vi "Pointer producer consumer Manual Motor Controls.vi"(0 "Iteraction Counter":u32, 1 "loopback":bool, 5 "Input Array":bool[](array[boolean]), 6 "Impulse IN":i32, 8 "Reverse moving":bool, 9 "PA°":u16 max=359, 11 "PA Correction°":dbl min=-26.3 max=26.3 step=0.1 format="%#_3g", 13 "No. Impulses":u8, 14 "Modulo num":u8) -> (3 "get info?":bool, 4 "PA rounded":dbl, 10 "Output Number":i32, 12 "Impulses":bool, 15 "Impulse OUT":i32)   [LabVIEW 2014]
panel:
  out "PA real":dbl
  out "Array Code IN":u32
  out "Output Command":string
  out "Array Code OUT":u32
  out "HEX Out Cmd":string=" "
  in  "error in (no error)":errorcluster
  out "Down":bool
  out "Left":bool
  out "Up":bool
  out "Right":bool
  # "Autobalance"
  # "Array code after angle transposition"
  # "Loopback"
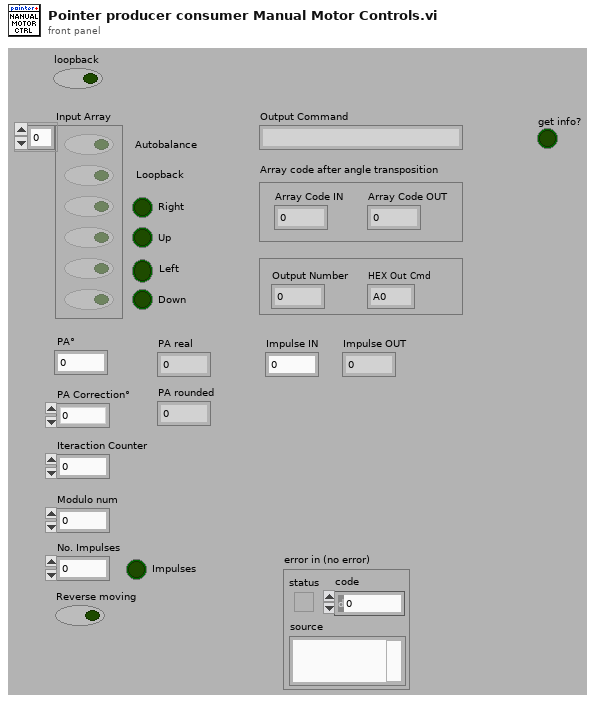
[diagram p1: front panel]
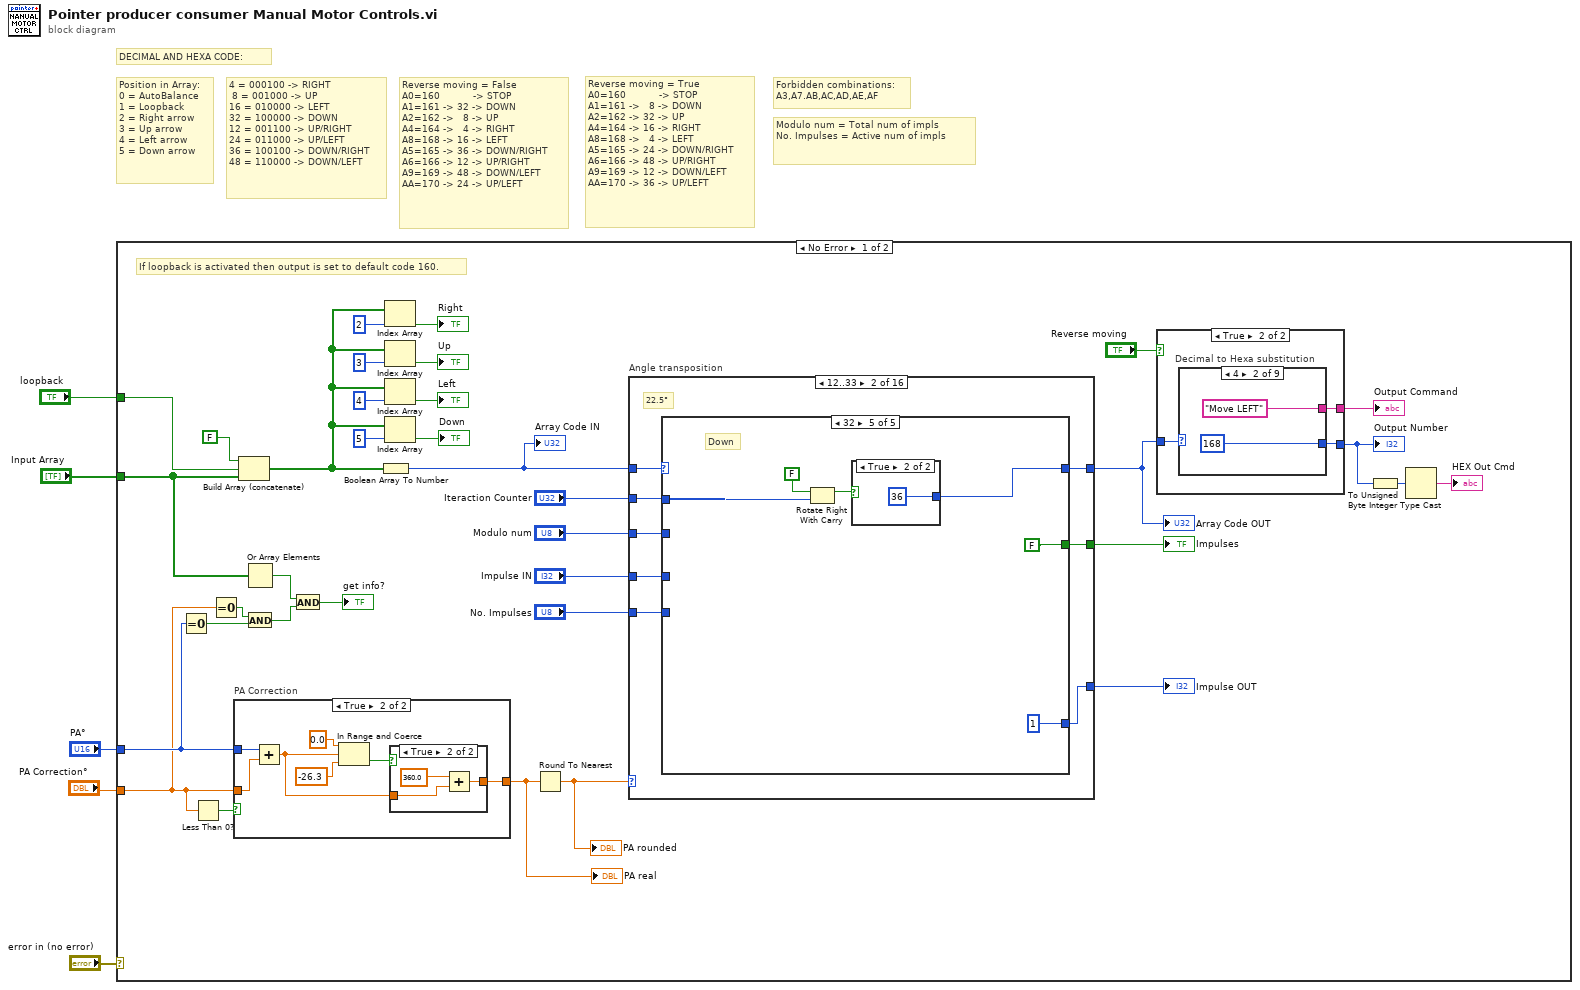
[diagram p0: block diagram]
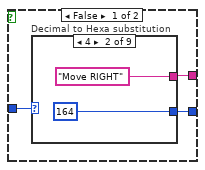
[diagram p2: hidden frame]
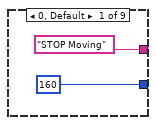
[diagram p3: hidden frame]
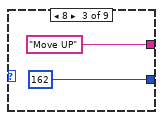
[diagram p4: hidden frame]
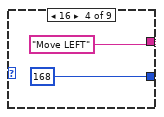
[diagram p5: hidden frame]
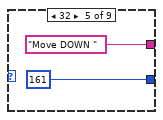
[diagram p6: hidden frame]
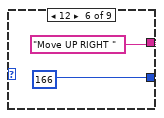
[diagram p7: hidden frame]
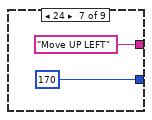
[diagram p8: hidden frame]
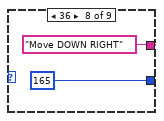
[diagram p9: hidden frame]
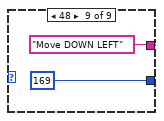
[diagram p10: hidden frame]
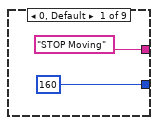
[diagram p11: hidden frame]
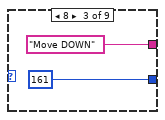
[diagram p12: hidden frame]
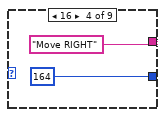
[diagram p13: hidden frame]
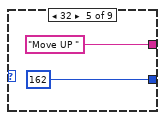
[diagram p14: hidden frame]
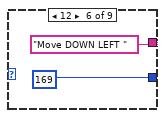
[diagram p15: hidden frame]
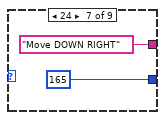
[diagram p16: hidden frame]
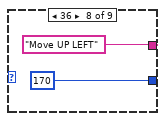
[diagram p17: hidden frame]
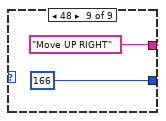
[diagram p18: hidden frame]
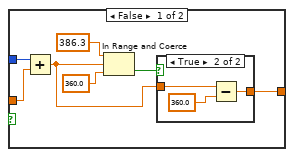
[diagram p19: hidden frame]
diagram:
  # "Reverse moving = True\nA0=160 \t\t        -> STOP\nA1=161 ->   8 -> DOWN\nA2=162 -> 32 -> UP\nA4=164 -> 16 -> RIGHT\nA8=168 ->   4 -> LEFT\nA5=165 -> 24 -> DOWN/RIGHT\nA6=166 -> 48 -> UP/RIGHT\nA9=169 -> 12 -> DOWN/LEFT\nAA=170 -> 36 -> UP/LEFT"
  # "Modulo num = Total num of impls \nNo. Impulses = Active num of impls"
  # "Position in Array: \n0 = AutoBalance\n1 = Loopback\n2 = Right arrow\n3 = Up arrow\n4 = Left arrow\n5 = Down arrow"
  # "4 = 000100 -> RIGHT\n 8 = 001000 -> UP \n16 = 010000 -> LEFT\n32 = 100000 -> DOWN\n12 = 001100 -> UP/RIGHT \n24 = 011000 -> UP/LEFT\n36 = 100100 -> DOWN/RIGHT\n48 = 110000 -> DOWN/LEFT"
  # "Forbidden combinations:\nA3,A7.AB,AC,AD,AE,AF"
  # "DECIMAL AND HEXA CODE:"
  # "Reverse moving = False\nA0=160 \t\t        -> STOP\nA1=161 -> 32 -> DOWN\nA2=162 ->   8 -> UP\nA4=164 ->   4 -> RIGHT\nA8=168 -> 16 -> LEFT\nA5=165 -> 36 -> DOWN/RIGHT\nA6=166 -> 12 -> UP/RIGHT\nA9=169 -> 48 -> DOWN/LEFT\nAA=170 -> 24 -> UP/LEFT"
  n1 = case shown="No Error" "error in (no error)" {
    tunnel: "PA°" -> [w15 _]
    tunnel: "PA Correction°" -> [w14 _]
    tunnel: "Input Array" -> [w11 _]
    tunnel: "loopback" -> [w6 _]
    frame No Error {
      # "If loopback is activated then output is set to default code 160."
      n2 = Equal To 0?(x=w15) -> (x = 0?=w7:bool)
      n3 = Less Than 0?(x=w14) -> (x < 0?=w25:bool)
      n4 = Equal To 0?(x=w14) -> (x = 0?=w8:bool)
      n5 = case "PA Correction" shown="True" w25 {
        tunnel: w15 -> [w84 w97]
        tunnel: [w85 w95] -> w23
        tunnel: w14 -> [w86 w96]
        frame False {
          n6 = Add(x=w84, y=w86) -> (x+y=w83:dbl)
          n7 = In Range and Coerce(upper limit=386.3, x=w83, lower limit=360.0) -> (In Range?=w87:bool)  [unwired: 1 out]
          n8 = case shown="True" w87 {
            tunnel: [w90 w93] -> w85
            tunnel: w83 -> [w90 w91]
            frame False {
            }
            frame True {
              n9 = Subtract(x=w91, y=360.0) -> (x-y=w93:dbl)
            }
          }
        }
        frame True {
          n10 = Add(x=w97, y=w96) -> (x+y=w98:dbl)
          n11 = In Range and Coerce(upper limit=0.0, x=w98, lower limit=-26.3) -> (In Range?=w94:bool)  [unwired: 1 out]
          n12 = case shown="True" w94 {
            tunnel: [w101 w104] -> w95
            tunnel: w98 -> [w101 w103]
            frame False {
            }
            frame True {
              n13 = Add(x=360.0 ("y"), y=w103) -> (x+y=w104:dbl)
            }
          }
        }
      }
      "PA real" <- w23
      n14 = Build Array (concatenate)(FALSE, w6, w11) -> (w12:bool[])
      n15 = Or Array Elements(Boolean array=w11) -> (logical OR=w10:bool)
      n16 = And(x=w8, y=w7) -> (x .and. y?=w9:bool)
      n17 = And(x=w10, y=w9) -> (x .and. y?=→"get info?":bool)
      n18 = Boolean Array To Number(Boolean array=w12) -> (number=w28:u32)
      "Array Code IN" <- w28
      n19 = Index Array(array=w12, index=2) -> (element=→"Right":bool)
      n20 = Index Array(array=w12, index=3) -> (element=→"Up":bool)
      n21 = Index Array(array=w12, index=4) -> (element=→"Left":bool)
      n22 = Index Array(array=w12, index=5) -> (element=→"Down":bool)
      n23 = Round To Nearest(number=w23) -> (nearest integer value=w21:dbl)
      "PA rounded" <- w21
      n24 = case "Angle transposition" shown="12..33" w21 {
        tunnel: w28 -> [w107 w114 w189 w202 w277 w291 w365 w379 w453 w467 w541 w555 w629 w643 w717 w731]
        tunnel: [w107 w115 w190 w203 w278 w289 w366 w377 w454 w465 w542 w553 w630 w641 w718 w729] -> w17
        tunnel: "Iteraction Counter" -> [_ w113 _ w201 _ w290 _ w378 _ w466 _ w554 _ w642 _ w730]
        tunnel: "Impulse IN" -> [_ w109 _ w197 _ w284 _ w373 _ w461 _ w548 _ w637 _ w724]
        tunnel: "Modulo num" -> [_ w110 _ w198 _ w286 _ w374 _ w462 _ w550 _ w636 _ w726]
        tunnel: "No. Impulses" -> [_ w108 _ w196 _ w285 _ w372 _ w460 _ w549 _ w638 _ w725]
        tunnel: [FALSE w112 FALSE w200 FALSE w288 FALSE w375 FALSE w463 FALSE w552 FALSE w640 FALSE w728] -> w26
        tunnel: [1 w111 1 w199 1 w287 1 w376 1 w464 1 w551 1 w639 1 w727] -> w24
        frame 0..11, 349..359, Default {
          # "0°"
        }
        frame 12..33 {
          # "22.5°"
          n25 = case shown="32" w114 {
            selector: w114 -> [w118 _ _ _ _]
            tunnel: [w118 w124 w147 w158 w181] -> w115
            tunnel: w113 -> [_ w125 w149 w155 w182]
            tunnel: [FALSE w123 FALSE w157 FALSE] -> w112
            tunnel: [1 w122 1 w159 1] -> w111
            tunnel: w110 -> [_ w119 _ w153 _]
            tunnel: w109 -> [_ w121 _ w156 _]
            tunnel: w108 -> [_ w120 _ w154 _]
            frame 0, Default {
            }
            frame 4 {
              (unwired) u8 7 ("Modulo num")
              (unwired) u8 8 ("Modulo num")
              # "Right"
              n26 = case "Decimal to Hexa substitution" shown="1, Default" w121 {
                tunnel: [TRUE FALSE] -> w133
                frame 1, Default {
                }
                frame 0 {
                }
              }
              n27 = case "Decimal to Hexa substitution" shown="1, Default" w121 {
                selector: w121 -> [w136 w138]
                tunnel: [w137 w138] -> w126
                frame 1, Default {
                  n28 = Increment(x=w136) -> (x+1=w137:i32)
                }
                frame 0 {
                }
              }
              n29 = Quotient & Remainder(x=w125, y=w119) -> (x-y*floor(x/y)=w135:u32)  [unwired: 1 out]
              n30 = Equal?(x=w135, y=0) -> (x = y?=w132:bool)
              n31 = Or(x=w132, y=w133) -> (x .or. y?=w123:bool)
              n32 = case shown="False" w123 {
                tunnel: [4 12] -> w124
                frame False {
                }
                frame True {
                }
              }
              n33 = case shown="True" w132 {
                tunnel: [1 w142] -> w131
                tunnel: w120 -> [_ w142]
                frame False {
                }
                frame True {
                }
              }
              n34 = Build Array(w131, w126) -> (w130:i32[])
              n35 = Sort 1D Array(array=w130) -> (sorted array=w129:i32[])
              n36 = Index Array(array=w129) -> (element #1=w128:i32, element #2=w127:i32)  [unwired: 2 in]
              n37 = Subtract(x=w127, y=w128) -> (x-y=w122:i32)
            }
            frame 8 {
              # "Up"
              n38 = Rotate Right With Carry(2:w149, 3:FALSE ("carry")) -> (1:w148:bool)  [unwired: 1 out]
              n39 = case shown="True" w148 {
                tunnel: [8 24] -> w147
                frame False {
                }
                frame True {
                }
              }
            }
            frame 16 {
              (unwired) u8 7 ("Modulo num")
              (unwired) u8 8 ("Modulo num")
              # "Left"
              n40 = case "Decimal to Hexa substitution" shown="1, Default" w156 {
                tunnel: [TRUE FALSE] -> w167
                frame 1, Default {
                }
                frame 0 {
                }
              }
              n41 = case "Decimal to Hexa substitution" shown="1, Default" w156 {
                selector: w156 -> [w170 w172]
                tunnel: [w171 w172] -> w160
                frame 1, Default {
                  n42 = Increment(x=w170) -> (x+1=w171:i32)
                }
                frame 0 {
                }
              }
              n43 = Quotient & Remainder(x=w155, y=w153) -> (x-y*floor(x/y)=w169:u32)  [unwired: 1 out]
              n44 = Equal?(x=w169, y=0) -> (x = y?=w166:bool)
              n45 = Or(x=w166, y=w167) -> (x .or. y?=w157:bool)
              n46 = case shown="True" w157 {
                tunnel: [16 48] -> w158
                frame False {
                }
                frame True {
                }
              }
              n47 = case shown="True" w166 {
                tunnel: [1 w176] -> w165
                tunnel: w154 -> [_ w176]
                frame False {
                }
                frame True {
                }
              }
              n48 = Build Array(w165, w160) -> (w164:i32[])
              n49 = Sort 1D Array(array=w164) -> (sorted array=w163:i32[])
              n50 = Index Array(array=w163) -> (element #1=w162:i32, element #2=w161:i32)  [unwired: 2 in]
              n51 = Subtract(x=w161, y=w162) -> (x-y=w159:i32)
            }
            frame 32 {
              # "Down"
              n52 = Rotate Right With Carry(2:w182, 3:FALSE ("carry")) -> (1:w183:bool)  [unwired: 1 out]
              n53 = case shown="True" w183 {
                tunnel: [32 36] -> w181
                frame False {
                }
                frame True {
                }
              }
            }
          }
        }
        frame 34..56 {
          # "45°"
          n54 = case shown="32" w189 {
            selector: w189 -> [w191 _ _ _ _]
            tunnel: [w191 12 24 48 36] -> w190
            frame 0, Default {
            }
            frame 4 {
              # "Right"
            }
            frame 8 {
              # "Up"
            }
            frame 16 {
              # "Left"
            }
            frame 32 {
              # "Down"
            }
          }
        }
        frame 57..78 {
          # "67.5°"
          n55 = case shown="8" w202 {
            selector: w202 -> [w206 _ _ _ _]
            tunnel: [w206 w209 w217 w243 w252] -> w203
            tunnel: w201 -> [_ w210 w220 w244 w253]
            tunnel: [FALSE FALSE w218 FALSE w251] -> w200
            tunnel: [1 1 w221 1 w255] -> w199
            tunnel: w198 -> [_ _ w215 _ w249]
            tunnel: w197 -> [_ _ w219 _ w254]
            tunnel: w196 -> [_ _ w216 _ w250]
            frame 0, Default {
            }
            frame 4 {
              # "Right"
              n56 = Rotate Right With Carry(2:w210, 3:FALSE ("carry")) -> (1:w211:bool)  [unwired: 1 out]
              n57 = case shown="False" w211 {
                tunnel: [8 12] -> w209
                frame False {
                }
                frame True {
                }
              }
            }
            frame 8 {
              (unwired) u8 7 ("Modulo num")
              (unwired) u8 8 ("Modulo num")
              # "Up"
              n58 = case "Decimal to Hexa substitution" shown="1, Default" w219 {
                tunnel: [TRUE FALSE] -> w229
                frame 1, Default {
                }
                frame 0 {
                }
              }
              n59 = case "Decimal to Hexa substitution" shown="1, Default" w219 {
                selector: w219 -> [w232 w234]
                tunnel: [w233 w234] -> w222
                frame 1, Default {
                  n60 = Increment(x=w232) -> (x+1=w233:i32)
                }
                frame 0 {
                }
              }
              n61 = Quotient & Remainder(x=w220, y=w215) -> (x-y*floor(x/y)=w231:u32)  [unwired: 1 out]
              n62 = Equal?(x=w231, y=0) -> (x = y?=w228:bool)
              n63 = Or(x=w228, y=w229) -> (x .or. y?=w218:bool)
              n64 = case shown="False" w218 {
                tunnel: [16 24] -> w217
                frame False {
                }
                frame True {
                }
              }
              n65 = case shown="True" w228 {
                tunnel: [1 w238] -> w227
                tunnel: w216 -> [_ w238]
                frame False {
                }
                frame True {
                }
              }
              n66 = Build Array(w227, w222) -> (w226:i32[])
              n67 = Sort 1D Array(array=w226) -> (sorted array=w225:i32[])
              n68 = Index Array(array=w225) -> (element #1=w224:i32, element #2=w223:i32)  [unwired: 2 in]
              n69 = Subtract(x=w223, y=w224) -> (x-y=w221:i32)
            }
            frame 16 {
              # "Left"
              n70 = Rotate Right With Carry(2:w244, 3:FALSE ("carry")) -> (1:w246:bool)  [unwired: 1 out]
              n71 = case shown="True" w246 {
                tunnel: [32 48] -> w243
                frame False {
                }
                frame True {
                }
              }
            }
            frame 32 {
              (unwired) u8 7 ("Modulo num")
              (unwired) u8 8 ("Modulo num")
              # "Down"
              n72 = case "Decimal to Hexa substitution" shown="1, Default" w254 {
                tunnel: [TRUE FALSE] -> w263
                frame 1, Default {
                }
                frame 0 {
                }
              }
              n73 = case "Decimal to Hexa substitution" shown="1, Default" w254 {
                selector: w254 -> [w266 w268]
                tunnel: [w267 w268] -> w256
                frame 1, Default {
                  n74 = Increment(x=w266) -> (x+1=w267:i32)
                }
                frame 0 {
                }
              }
              n75 = Quotient & Remainder(x=w253, y=w249) -> (x-y*floor(x/y)=w265:u32)  [unwired: 1 out]
              n76 = Equal?(x=w265, y=0) -> (x = y?=w262:bool)
              n77 = Or(x=w262, y=w263) -> (x .or. y?=w251:bool)
              n78 = case shown="True" w251 {
                tunnel: [4 36] -> w252
                frame False {
                }
                frame True {
                }
              }
              n79 = case shown="True" w262 {
                tunnel: [1 w272] -> w261
                tunnel: w250 -> [_ w272]
                frame False {
                }
                frame True {
                }
              }
              n80 = Build Array(w261, w256) -> (w260:i32[])
              n81 = Sort 1D Array(array=w260) -> (sorted array=w259:i32[])
              n82 = Index Array(array=w259) -> (element #1=w258:i32, element #2=w257:i32)  [unwired: 2 in]
              n83 = Subtract(x=w257, y=w258) -> (x-y=w255:i32)
            }
          }
        }
        frame 79..101 {
          # "90°"
          n84 = case shown="8" w277 {
            selector: w277 -> [w279 _ _ _ _]
            tunnel: [w279 8 16 32 4] -> w278
            frame 0, Default {
            }
            frame 4 {
              # "Right"
            }
            frame 8 {
              # "Up"
            }
            frame 16 {
              # "Left"
            }
            frame 32 {
              # "Down"
            }
          }
        }
        frame 102..123 {
          # "112.5°"
          n85 = case shown="32" w291 {
            selector: w291 -> [w294 _ _ _ _]
            tunnel: [w294 w297 w308 w331 w339] -> w289
            tunnel: w290 -> [_ w298 w309 w332 w343]
            tunnel: [FALSE FALSE w307 FALSE w340] -> w288
            tunnel: [1 1 w306 1 w341] -> w287
            tunnel: w286 -> [_ _ w303 _ w337]
            tunnel: w285 -> [_ _ w304 _ w338]
            tunnel: w284 -> [_ _ w305 _ w342]
            frame 0, Default {
            }
            frame 4 {
              # "Right"
              n86 = Rotate Right With Carry(2:w298, 3:FALSE ("carry")) -> (1:w300:bool)  [unwired: 1 out]
              n87 = case shown="True" w300 {
                tunnel: [8 24] -> w297
                frame False {
                }
                frame True {
                }
              }
            }
            frame 8 {
              (unwired) u8 7 ("Modulo num")
              (unwired) u8 8 ("Modulo num")
              # "Up"
              n88 = case "Decimal to Hexa substitution" shown="1, Default" w305 {
                tunnel: [TRUE FALSE] -> w317
                frame 1, Default {
                }
                frame 0 {
                }
              }
              n89 = case "Decimal to Hexa substitution" shown="1, Default" w305 {
                selector: w305 -> [w320 w322]
                tunnel: [w321 w322] -> w310
                frame 1, Default {
                  n90 = Increment(x=w320) -> (x+1=w321:i32)
                }
                frame 0 {
                }
              }
              n91 = Quotient & Remainder(x=w309, y=w303) -> (x-y*floor(x/y)=w319:u32)  [unwired: 1 out]
              n92 = Equal?(x=w319, y=0) -> (x = y?=w316:bool)
              n93 = Or(x=w316, y=w317) -> (x .or. y?=w307:bool)
              n94 = case shown="True" w307 {
                tunnel: [16 48] -> w308
                frame False {
                }
                frame True {
                }
              }
              n95 = case shown="True" w316 {
                tunnel: [1 w326] -> w315
                tunnel: w304 -> [_ w326]
                frame False {
                }
                frame True {
                }
              }
              n96 = Build Array(w315, w310) -> (w314:i32[])
              n97 = Sort 1D Array(array=w314) -> (sorted array=w313:i32[])
              n98 = Index Array(array=w313) -> (element #1=w312:i32, element #2=w311:i32)  [unwired: 2 in]
              n99 = Subtract(x=w311, y=w312) -> (x-y=w306:i32)
            }
            frame 16 {
              # "Left"
              n100 = Rotate Right With Carry(2:w332, 3:FALSE ("carry")) -> (1:w333:bool)  [unwired: 1 out]
              n101 = case shown="False" w333 {
                tunnel: [32 36] -> w331
                frame False {
                }
                frame True {
                }
              }
            }
            frame 32 {
              (unwired) u8 7 ("Modulo num")
              (unwired) u8 8 ("Modulo num")
              # "Down"
              n102 = case "Decimal to Hexa substitution" shown="1, Default" w342 {
                tunnel: [TRUE FALSE] -> w351
                frame 1, Default {
                }
                frame 0 {
                }
              }
              n103 = case "Decimal to Hexa substitution" shown="1, Default" w342 {
                selector: w342 -> [w354 w356]
                tunnel: [w355 w356] -> w344
                frame 1, Default {
                  n104 = Increment(x=w354) -> (x+1=w355:i32)
                }
                frame 0 {
                }
              }
              n105 = Quotient & Remainder(x=w343, y=w337) -> (x-y*floor(x/y)=w353:u32)  [unwired: 1 out]
              n106 = Equal?(x=w353, y=0) -> (x = y?=w350:bool)
              n107 = Or(x=w350, y=w351) -> (x .or. y?=w340:bool)
              n108 = case shown="True" w340 {
                tunnel: [4 12] -> w339
                frame False {
                }
                frame True {
                }
              }
              n109 = case shown="True" w350 {
                tunnel: [1 w360] -> w349
                tunnel: w338 -> [_ w360]
                frame False {
                }
                frame True {
                }
              }
              n110 = Build Array(w349, w344) -> (w348:i32[])
              n111 = Sort 1D Array(array=w348) -> (sorted array=w347:i32[])
              n112 = Index Array(array=w347) -> (element #1=w346:i32, element #2=w345:i32)  [unwired: 2 in]
              n113 = Subtract(x=w345, y=w346) -> (x-y=w341:i32)
            }
          }
        }
        frame 124..146 {
          # "135°"
          n114 = case shown="32" w365 {
            selector: w365 -> [w367 _ _ _ _]
            tunnel: [w367 24 48 36 12] -> w366
            frame 0, Default {
            }
            frame 4 {
            }
            frame 8 {
            }
            frame 16 {
            }
            frame 32 {
            }
          }
        }
        frame 147..168 {
          # "157.5°"
          n115 = case shown="4" w379 {
            selector: w379 -> [w382 _ _ _ _]
            tunnel: [w382 w386 w411 w422 w445] -> w377
            tunnel: w378 -> [_ w389 w413 w423 w446]
            tunnel: [1 w385 1 w420 1] -> w376
            tunnel: [FALSE w387 FALSE w421 FALSE] -> w375
            tunnel: w374 -> [_ w383 _ w417 _]
            tunnel: w373 -> [_ w388 _ w419 _]
            tunnel: w372 -> [_ w384 _ w418 _]
            frame 0, Default {
            }
            frame 4 {
              (unwired) u8 7 ("Modulo num")
              (unwired) u8 8 ("Modulo num")
              # "Right"
              n116 = case "Decimal to Hexa substitution" shown="1, Default" w388 {
                tunnel: [TRUE FALSE] -> w397
                frame 1, Default {
                }
                frame 0 {
                }
              }
              n117 = case "Decimal to Hexa substitution" shown="1, Default" w388 {
                selector: w388 -> [w400 w402]
                tunnel: [w401 w402] -> w390
                frame 1, Default {
                  n118 = Increment(x=w400) -> (x+1=w401:i32)
                }
                frame 0 {
                }
              }
              n119 = Quotient & Remainder(x=w389, y=w383) -> (x-y*floor(x/y)=w399:u32)  [unwired: 1 out]
              n120 = Equal?(x=w399, y=0) -> (x = y?=w396:bool)
              n121 = Or(x=w396, y=w397) -> (x .or. y?=w387:bool)
              n122 = case shown="True" w387 {
                tunnel: [16 24] -> w386
                frame False {
                }
                frame True {
                }
              }
              n123 = case shown="False" w396 {
                tunnel: [1 w406] -> w395
                tunnel: w384 -> [_ w406]
                frame False {
                }
                frame True {
                }
              }
              n124 = Build Array(w395, w390) -> (w394:i32[])
              n125 = Sort 1D Array(array=w394) -> (sorted array=w393:i32[])
              n126 = Index Array(array=w393) -> (element #1=w392:i32, element #2=w391:i32)  [unwired: 2 in]
              n127 = Subtract(x=w391, y=w392) -> (x-y=w385:i32)
            }
            frame 8 {
              # "Up"
              n128 = Rotate Right With Carry(2:w413, 3:FALSE ("carry")) -> (1:w412:bool)  [unwired: 1 out]
              n129 = case shown="False" w412 {
                tunnel: [32 48] -> w411
                frame False {
                }
                frame True {
                }
              }
            }
            frame 16 {
              (unwired) u8 8 ("Modulo num")
              (unwired) u8 7 ("Modulo num")
              # "Left"
              n130 = case "Decimal to Hexa substitution" shown="1, Default" w419 {
                tunnel: [TRUE FALSE] -> w431
                frame 1, Default {
                }
                frame 0 {
                }
              }
              n131 = case "Decimal to Hexa substitution" shown="1, Default" w419 {
                selector: w419 -> [w434 w436]
                tunnel: [w435 w436] -> w424
                frame 1, Default {
                  n132 = Increment(x=w434) -> (x+1=w435:i32)
                }
                frame 0 {
                }
              }
              n133 = Quotient & Remainder(x=w423, y=w417) -> (x-y*floor(x/y)=w433:u32)  [unwired: 1 out]
              n134 = Equal?(x=w433, y=0) -> (x = y?=w430:bool)
              n135 = Or(x=w430, y=w431) -> (x .or. y?=w421:bool)
              n136 = case shown="True" w421 {
                tunnel: [4 36] -> w422
                frame False {
                }
                frame True {
                }
              }
              n137 = case shown="False" w430 {
                tunnel: [1 w440] -> w429
                tunnel: w418 -> [_ w440]
                frame False {
                }
                frame True {
                }
              }
              n138 = Build Array(w429, w424) -> (w428:i32[])
              n139 = Sort 1D Array(array=w428) -> (sorted array=w427:i32[])
              n140 = Index Array(array=w427) -> (element #1=w426:i32, element #2=w425:i32)  [unwired: 2 in]
              n141 = Subtract(x=w425, y=w426) -> (x-y=w420:i32)
            }
            frame 32 {
              # "Down"
              n142 = Rotate Right With Carry(2:w446, 3:FALSE ("carry")) -> (1:w447:bool)  [unwired: 1 out]
              n143 = case shown="False" w447 {
                tunnel: [8 12] -> w445
                frame False {
                }
                frame True {
                }
              }
            }
          }
        }
        frame 169..191 {
          # "180°"
          n144 = case shown="32" w453 {
            selector: w453 -> [w455 _ _ _ _]
            tunnel: [w455 16 32 4 8] -> w454
            frame 0, Default {
            }
            frame 4 {
            }
            frame 8 {
            }
            frame 16 {
            }
            frame 32 {
            }
          }
        }
        frame 192..213 {
          # "202.5°"
          n145 = case shown="16" w467 {
            selector: w467 -> [w470 _ _ _ _]
            tunnel: [w470 w474 w499 w507 w533] -> w465
            tunnel: w466 -> [_ w477 w501 w509 w534]
            tunnel: [1 w473 1 w511 1] -> w464
            tunnel: [FALSE w475 FALSE w508 FALSE] -> w463
            tunnel: w462 -> [_ w471 _ w505 _]
            tunnel: w461 -> [_ w476 _ w510 _]
            tunnel: w460 -> [_ w472 _ w506 _]
            frame 0, Default {
            }
            frame 4 {
              (unwired) u8 7 ("Modulo num")
              (unwired) u8 8 ("Modulo num")
              # "Right"
              n146 = case "Decimal to Hexa substitution" shown="1, Default" w476 {
                tunnel: [TRUE FALSE] -> w485
                frame 1, Default {
                }
                frame 0 {
                }
              }
              n147 = case "Decimal to Hexa substitution" shown="1, Default" w476 {
                selector: w476 -> [w488 w490]
                tunnel: [w489 w490] -> w478
                frame 1, Default {
                  n148 = Increment(x=w488) -> (x+1=w489:i32)
                }
                frame 0 {
                }
              }
              n149 = Quotient & Remainder(x=w477, y=w471) -> (x-y*floor(x/y)=w487:u32)  [unwired: 1 out]
              n150 = Equal?(x=w487, y=0) -> (x = y?=w484:bool)
              n151 = Or(x=w484, y=w485) -> (x .or. y?=w475:bool)
              n152 = case shown="False" w475 {
                tunnel: [16 48] -> w474
                frame False {
                }
                frame True {
                }
              }
              n153 = case shown="False" w484 {
                tunnel: [1 w494] -> w483
                tunnel: w472 -> [_ w494]
                frame False {
                }
                frame True {
                }
              }
              n154 = Build Array(w483, w478) -> (w482:i32[])
              n155 = Sort 1D Array(array=w482) -> (sorted array=w481:i32[])
              n156 = Index Array(array=w481) -> (element #1=w480:i32, element #2=w479:i32)  [unwired: 2 in]
              n157 = Subtract(x=w479, y=w480) -> (x-y=w473:i32)
            }
            frame 8 {
              # "Up"
              n158 = Rotate Right With Carry(2:w501, 3:FALSE ("carry")) -> (1:w500:bool)  [unwired: 1 out]
              n159 = case shown="True" w500 {
                tunnel: [32 36] -> w499
                frame False {
                }
                frame True {
                }
              }
            }
            frame 16 {
              (unwired) u8 7 ("Modulo num")
              (unwired) u8 8 ("Modulo num")
              # "Left"
              n160 = case "Decimal to Hexa substitution" shown="1, Default" w510 {
                tunnel: [TRUE FALSE] -> w519
                frame 1, Default {
                }
                frame 0 {
                }
              }
              n161 = case "Decimal to Hexa substitution" shown="1, Default" w510 {
                selector: w510 -> [w522 w524]
                tunnel: [w523 w524] -> w512
                frame 1, Default {
                  n162 = Increment(x=w522) -> (x+1=w523:i32)
                }
                frame 0 {
                }
              }
              n163 = Quotient & Remainder(x=w509, y=w505) -> (x-y*floor(x/y)=w521:u32)  [unwired: 1 out]
              n164 = Equal?(x=w521, y=0) -> (x = y?=w518:bool)
              n165 = Or(x=w518, y=w519) -> (x .or. y?=w508:bool)
              n166 = case shown="False" w508 {
                tunnel: [4 12] -> w507
                frame False {
                }
                frame True {
                }
              }
              n167 = case shown="False" w518 {
                tunnel: [1 w528] -> w517
                tunnel: w506 -> [_ w528]
                frame False {
                }
                frame True {
                }
              }
              n168 = Build Array(w517, w512) -> (w516:i32[])
              n169 = Sort 1D Array(array=w516) -> (sorted array=w515:i32[])
              n170 = Index Array(array=w515) -> (element #1=w514:i32, element #2=w513:i32)  [unwired: 2 in]
              n171 = Subtract(x=w513, y=w514) -> (x-y=w511:i32)
            }
            frame 32 {
              # "Down"
              n172 = Rotate Right With Carry(2:w534, 3:FALSE ("carry")) -> (1:w535:bool)  [unwired: 1 out]
              n173 = case shown="True" w535 {
                tunnel: [8 24] -> w533
                frame False {
                }
                frame True {
                }
              }
            }
          }
        }
        frame 214..236 {
          # "225°"
          n174 = case shown="32" w541 {
            selector: w541 -> [w543 _ _ _ _]
            tunnel: [w543 48 36 12 24] -> w542
            frame 0, Default {
            }
            frame 4 {
            }
            frame 8 {
            }
            frame 16 {
            }
            frame 32 {
            }
          }
        }
        frame 237..258 {
          # "247.5°"
          n175 = case shown="32" w555 {
            selector: w555 -> [w558 _ _ _ _]
            tunnel: [w558 w561 w570 w595 w604] -> w553
            tunnel: w554 -> [_ w562 w571 w596 w607]
            tunnel: [FALSE FALSE w569 FALSE w605] -> w552
            tunnel: [1 1 w573 1 w603] -> w551
            tunnel: w550 -> [_ _ w567 _ w601]
            tunnel: w549 -> [_ _ w568 _ w602]
            tunnel: w548 -> [_ _ w572 _ w606]
            frame 0, Default {
            }
            frame 4 {
              # "Right"
              n176 = Rotate Right With Carry(2:w562, 3:FALSE ("carry")) -> (1:w564:bool)  [unwired: 1 out]
              n177 = case shown="False" w564 {
                tunnel: [32 48] -> w561
                frame False {
                }
                frame True {
                }
              }
            }
            frame 8 {
              (unwired) u8 7 ("Modulo num")
              (unwired) u8 8 ("Modulo num")
              # "Up"
              n178 = case "Decimal to Hexa substitution" shown="1, Default" w572 {
                tunnel: [TRUE FALSE] -> w581
                frame 1, Default {
                }
                frame 0 {
                }
              }
              n179 = case "Decimal to Hexa substitution" shown="1, Default" w572 {
                selector: w572 -> [w584 w586]
                tunnel: [w585 w586] -> w574
                frame 1, Default {
                  n180 = Increment(x=w584) -> (x+1=w585:i32)
                }
                frame 0 {
                }
              }
              n181 = Quotient & Remainder(x=w571, y=w567) -> (x-y*floor(x/y)=w583:u32)  [unwired: 1 out]
              n182 = Equal?(x=w583, y=0) -> (x = y?=w580:bool)
              n183 = Or(x=w580, y=w581) -> (x .or. y?=w569:bool)
              n184 = case shown="False" w569 {
                tunnel: [4 36] -> w570
                frame False {
                }
                frame True {
                }
              }
              n185 = case shown="True" w580 {
                tunnel: [1 w590] -> w579
                tunnel: w568 -> [_ w590]
                frame False {
                }
                frame True {
                }
              }
              n186 = Build Array(w579, w574) -> (w578:i32[])
              n187 = Sort 1D Array(array=w578) -> (sorted array=w577:i32[])
              n188 = Index Array(array=w577) -> (element #1=w576:i32, element #2=w575:i32)  [unwired: 2 in]
              n189 = Subtract(x=w575, y=w576) -> (x-y=w573:i32)
            }
            frame 16 {
              # "Left"
              n190 = Rotate Right With Carry(2:w596, 3:FALSE ("carry")) -> (1:w597:bool)  [unwired: 1 out]
              n191 = case shown="False" w597 {
                tunnel: [8 12] -> w595
                frame False {
                }
                frame True {
                }
              }
            }
            frame 32 {
              (unwired) u8 7 ("Modulo num")
              (unwired) u8 8 ("Modulo num")
              # "Down"
              n192 = case "Decimal to Hexa substitution" shown="1, Default" w606 {
                tunnel: [TRUE FALSE] -> w615
                frame 1, Default {
                }
                frame 0 {
                }
              }
              n193 = case "Decimal to Hexa substitution" shown="1, Default" w606 {
                selector: w606 -> [w618 w620]
                tunnel: [w619 w620] -> w608
                frame 1, Default {
                  n194 = Increment(x=w618) -> (x+1=w619:i32)
                }
                frame 0 {
                }
              }
              n195 = Quotient & Remainder(x=w607, y=w601) -> (x-y*floor(x/y)=w617:u32)  [unwired: 1 out]
              n196 = Equal?(x=w617, y=0) -> (x = y?=w614:bool)
              n197 = Or(x=w614, y=w615) -> (x .or. y?=w605:bool)
              n198 = case shown="True" w605 {
                tunnel: [16 24] -> w604
                frame False {
                }
                frame True {
                }
              }
              n199 = case shown="True" w614 {
                tunnel: [1 w624] -> w613
                tunnel: w602 -> [_ w624]
                frame False {
                }
                frame True {
                }
              }
              n200 = Build Array(w613, w608) -> (w612:i32[])
              n201 = Sort 1D Array(array=w612) -> (sorted array=w611:i32[])
              n202 = Index Array(array=w611) -> (element #1=w610:i32, element #2=w609:i32)  [unwired: 2 in]
              n203 = Subtract(x=w609, y=w610) -> (x-y=w603:i32)
            }
          }
        }
        frame 259..281 {
          # "270°"
          n204 = case shown="32" w629 {
            selector: w629 -> [w631 _ _ _ _]
            tunnel: [w631 32 4 8 16] -> w630
            frame 0, Default {
            }
            frame 4 {
            }
            frame 8 {
            }
            frame 16 {
            }
            frame 32 {
            }
          }
        }
        frame 282..303 {
          # "292.5°"
          n205 = case shown="4" w643 {
            selector: w643 -> [w646 _ _ _ _]
            tunnel: [w646 w649 w660 w683 w693] -> w641
            tunnel: w642 -> [_ w650 w657 w684 w691]
            tunnel: [FALSE FALSE w659 FALSE w694] -> w640
            tunnel: [1 1 w661 1 w695] -> w639
            tunnel: w638 -> [_ _ w656 _ w690]
            tunnel: w637 -> [_ _ w658 _ w692]
            tunnel: w636 -> [_ _ w655 _ w689]
            frame 0, Default {
            }
            frame 4 {
              # "Right"
              n206 = Rotate Right With Carry(2:w650, 3:FALSE ("carry")) -> (1:w652:bool)  [unwired: 1 out]
              n207 = case shown="False" w652 {
                tunnel: [32 36] -> w649
                frame False {
                }
                frame True {
                }
              }
            }
            frame 8 {
              (unwired) u8 7 ("Modulo num")
              (unwired) u8 8 ("Modulo num")
              # "Up"
              n208 = case "Decimal to Hexa substitution" shown="1, Default" w658 {
                tunnel: [TRUE FALSE] -> w669
                frame 1, Default {
                }
                frame 0 {
                }
              }
              n209 = case "Decimal to Hexa substitution" shown="1, Default" w658 {
                selector: w658 -> [w672 w674]
                tunnel: [w673 w674] -> w662
                frame 1, Default {
                  n210 = Increment(x=w672) -> (x+1=w673:i32)
                }
                frame 0 {
                }
              }
              n211 = Quotient & Remainder(x=w657, y=w655) -> (x-y*floor(x/y)=w671:u32)  [unwired: 1 out]
              n212 = Equal?(x=w671, y=0) -> (x = y?=w668:bool)
              n213 = Or(x=w668, y=w669) -> (x .or. y?=w659:bool)
              n214 = case shown="True" w659 {
                tunnel: [4 12] -> w660
                frame False {
                }
                frame True {
                }
              }
              n215 = case shown="True" w668 {
                tunnel: [1 w678] -> w667
                tunnel: w656 -> [_ w678]
                frame False {
                }
                frame True {
                }
              }
              n216 = Build Array(w667, w662) -> (w666:i32[])
              n217 = Sort 1D Array(array=w666) -> (sorted array=w665:i32[])
              n218 = Index Array(array=w665) -> (element #1=w664:i32, element #2=w663:i32)  [unwired: 2 in]
              n219 = Subtract(x=w663, y=w664) -> (x-y=w661:i32)
            }
            frame 16 {
              # "Left"
              n220 = Rotate Right With Carry(2:w684, 3:FALSE ("carry")) -> (1:w685:bool)  [unwired: 1 out]
              n221 = case shown="True" w685 {
                tunnel: [8 24] -> w683
                frame False {
                }
                frame True {
                }
              }
            }
            frame 32 {
              (unwired) u8 7 ("Modulo num")
              (unwired) u8 8 ("Modulo num")
              # "Down"
              n222 = case "Decimal to Hexa substitution" shown="1, Default" w692 {
                tunnel: [TRUE FALSE] -> w703
                frame 1, Default {
                }
                frame 0 {
                }
              }
              n223 = case "Decimal to Hexa substitution" shown="1, Default" w692 {
                selector: w692 -> [w706 w708]
                tunnel: [w707 w708] -> w696
                frame 1, Default {
                  n224 = Increment(x=w706) -> (x+1=w707:i32)
                }
                frame 0 {
                }
              }
              n225 = Quotient & Remainder(x=w691, y=w689) -> (x-y*floor(x/y)=w705:u32)  [unwired: 1 out]
              n226 = Equal?(x=w705, y=0) -> (x = y?=w702:bool)
              n227 = Or(x=w702, y=w703) -> (x .or. y?=w694:bool)
              n228 = case shown="True" w694 {
                tunnel: [16 48] -> w693
                frame False {
                }
                frame True {
                }
              }
              n229 = case shown="True" w702 {
                tunnel: [1 w712] -> w701
                tunnel: w690 -> [_ w712]
                frame False {
                }
                frame True {
                }
              }
              n230 = Build Array(w701, w696) -> (w700:i32[])
              n231 = Sort 1D Array(array=w700) -> (sorted array=w699:i32[])
              n232 = Index Array(array=w699) -> (element #1=w698:i32, element #2=w697:i32)  [unwired: 2 in]
              n233 = Subtract(x=w697, y=w698) -> (x-y=w695:i32)
            }
          }
        }
        frame 304..326 {
          # "315°"
          n234 = case shown="4" w717 {
            selector: w717 -> [w719 _ _ _ _]
            tunnel: [w719 36 12 24 48] -> w718
            frame 0, Default {
            }
            frame 4 {
            }
            frame 8 {
            }
            frame 16 {
            }
            frame 32 {
            }
          }
        }
        frame 327..348 {
          # "337.5°"
          n235 = case shown="4" w731 {
            selector: w731 -> [w734 _ _ _ _]
            tunnel: [w734 w739 w763 w774 w797] -> w729
            tunnel: w730 -> [_ w741 w765 w775 w798]
            tunnel: [FALSE w738 FALSE w773 FALSE] -> w728
            tunnel: [1 w737 1 w772 1] -> w727
            tunnel: w726 -> [_ w735 _ w769 _]
            tunnel: w725 -> [_ w736 _ w770 _]
            tunnel: w724 -> [_ w740 _ w771 _]
            frame 0, Default {
            }
            frame 4 {
              (unwired) u8 7 ("Modulo num")
              (unwired) u8 8 ("Modulo num")
              # "Right"
              n236 = case "Decimal to Hexa substitution" shown="1, Default" w740 {
                tunnel: [TRUE FALSE] -> w749
                frame 1, Default {
                }
                frame 0 {
                }
              }
              n237 = case "Decimal to Hexa substitution" shown="1, Default" w740 {
                selector: w740 -> [w752 w754]
                tunnel: [w753 w754] -> w742
                frame 1, Default {
                  n238 = Increment(x=w752) -> (x+1=w753:i32)
                }
                frame 0 {
                }
              }
              n239 = Quotient & Remainder(x=w741, y=w735) -> (x-y*floor(x/y)=w751:u32)  [unwired: 1 out]
              n240 = Equal?(x=w751, y=0) -> (x = y?=w748:bool)
              n241 = Or(x=w748, y=w749) -> (x .or. y?=w738:bool)
              n242 = case shown="False" w738 {
                tunnel: [4 36] -> w739
                frame False {
                }
                frame True {
                }
              }
              n243 = case shown="False" w748 {
                tunnel: [1 w758] -> w747
                tunnel: w736 -> [_ w758]
                frame False {
                }
                frame True {
                }
              }
              n244 = Build Array(w747, w742) -> (w746:i32[])
              n245 = Sort 1D Array(array=w746) -> (sorted array=w745:i32[])
              n246 = Index Array(array=w745) -> (element #1=w744:i32, element #2=w743:i32)  [unwired: 2 in]
              n247 = Subtract(x=w743, y=w744) -> (x-y=w737:i32)
            }
            frame 8 {
              # "Up"
              n248 = Rotate Right With Carry(2:w765, 3:FALSE ("carry")) -> (1:w764:bool)  [unwired: 1 out]
              n249 = case shown="False" w764 {
                tunnel: [8 12] -> w763
                frame False {
                }
                frame True {
                }
              }
            }
            frame 16 {
              (unwired) u8 7 ("Modulo num")
              (unwired) u8 8 ("Modulo num")
              # "Left"
              n250 = case "Decimal to Hexa substitution" shown="1, Default" w771 {
                tunnel: [TRUE FALSE] -> w783
                frame 1, Default {
                }
                frame 0 {
                }
              }
              n251 = case "Decimal to Hexa substitution" shown="1, Default" w771 {
                selector: w771 -> [w786 w788]
                tunnel: [w787 w788] -> w776
                frame 1, Default {
                  n252 = Increment(x=w786) -> (x+1=w787:i32)
                }
                frame 0 {
                }
              }
              n253 = Quotient & Remainder(x=w775, y=w769) -> (x-y*floor(x/y)=w785:u32)  [unwired: 1 out]
              n254 = Equal?(x=w785, y=0) -> (x = y?=w782:bool)
              n255 = Or(x=w782, y=w783) -> (x .or. y?=w773:bool)
              n256 = case shown="True" w773 {
                tunnel: [16 24] -> w774
                frame False {
                }
                frame True {
                }
              }
              n257 = case shown="False" w782 {
                tunnel: [1 w792] -> w781
                tunnel: w770 -> [_ w792]
                frame False {
                }
                frame True {
                }
              }
              n258 = Build Array(w781, w776) -> (w780:i32[])
              n259 = Sort 1D Array(array=w780) -> (sorted array=w779:i32[])
              n260 = Index Array(array=w779) -> (element #1=w778:i32, element #2=w777:i32)  [unwired: 2 in]
              n261 = Subtract(x=w777, y=w778) -> (x-y=w772:i32)
            }
            frame 32 {
              # "Down"
              n262 = Rotate Right With Carry(2:w798, 3:FALSE ("carry")) -> (1:w799:bool)  [unwired: 1 out]
              n263 = case shown="True" w799 {
                tunnel: [32 48] -> w797
                frame False {
                }
                frame True {
                }
              }
            }
          }
        }
      }
      "Array Code OUT" <- w17
      "Impulse OUT" <- w24
      "Impulses" <- w26
      n264 = case shown="True" "Reverse moving" {
        tunnel: w17 -> [w43 w62]
        tunnel: [w42 w63] -> w20
        tunnel: [w41 w64] -> w19
        frame False {
          n265 = case "Decimal to Hexa substitution" shown="4" w43 {
            tunnel: ["STOP Moving" "Move RIGHT" "Move UP" "Move LEFT" "Move DOWN " "Move UP RIGHT " "Move UP LEFT" "Move DOWN RIGHT" "Move DOWN LEFT"] -> w41
            tunnel: [160 164 162 168 161 166 170 165 169] -> w42
            frame 0, Default {
            }
            frame 4 {
            }
            frame 8 {
            }
            frame 16 {
            }
            frame 32 {
            }
            frame 12 {
            }
            frame 24 {
            }
            frame 36 {
            }
            frame 48 {
            }
          }
        }
        frame True {
          n266 = case "Decimal to Hexa substitution" shown="4" w62 {
            tunnel: ["STOP Moving" "Move LEFT" "Move DOWN" "Move RIGHT" "Move UP " "Move DOWN LEFT " "Move DOWN RIGHT" "Move UP LEFT" "Move UP RIGHT"] -> w64
            tunnel: [160 168 161 164 162 169 165 170 166] -> w63
            frame 0, Default {
            }
            frame 4 {
            }
            frame 8 {
            }
            frame 16 {
            }
            frame 32 {
            }
            frame 12 {
            }
            frame 24 {
            }
            frame 36 {
            }
            frame 48 {
            }
          }
        }
      }
      "Output Number" <- w20
      "Output Command" <- w19
      n267 = To Unsigned Byte Integer(number=w20) -> (unsigned 8bit integer=w32:u8)
      n268 = Type Cast(x=w32) -> (*(type *) &x=→"HEX Out Cmd":string)  [unwired: 1 in]
    }
    frame Error {
    }
  }
